vi "Get Subtype Description.vi"(8 "error in (no error)":errorcluster, 11 "Keyboard Action in":refnum<class "Keyboard Action.lvclass">) -> (0 "error out":errorcluster, 2 "Subtype Description":string, 3 "Keyboard Action out":refnum<class "Keyboard Action.lvclass">)   [LabVIEW 2020, in "MacroAssert.lvlib" / "Keyboard Action.lvclass"]
doc: "Gets the subtype description for <B>Step in</B>, which describes what the step's subtype does specifically."
uses:
  Keyboard Action.lvclass
  Keyboard Action.lvclass/Keyboard Action.ctl
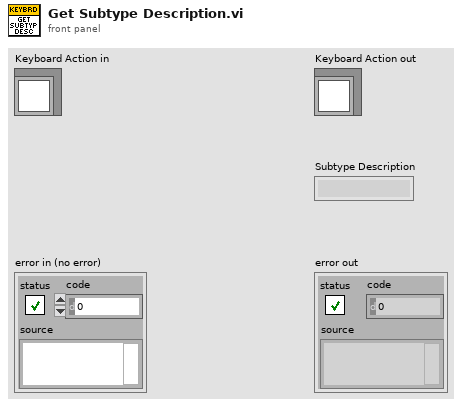
[diagram p1: front panel]
types:
  T1 = typedef "MacroAssert.lvlib/Keyboard Action.lvclass/Keyboard Action Type.ctl" = enum16{"Key Press", "Key Down", "Key Up", "Key Sequence"}
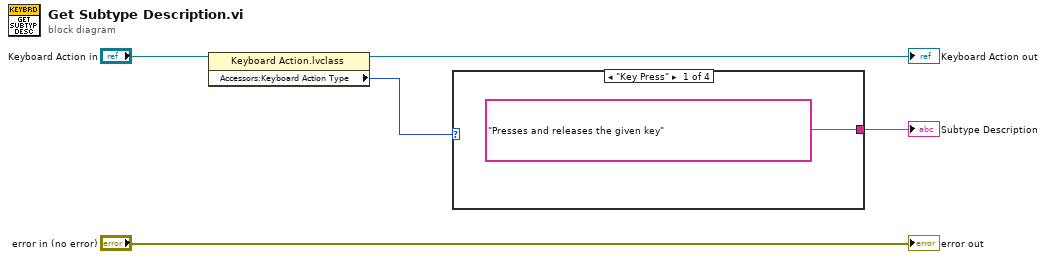
[diagram p0: block diagram]
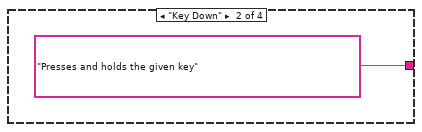
[diagram p2: hidden frame]
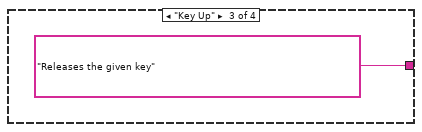
[diagram p3: hidden frame]
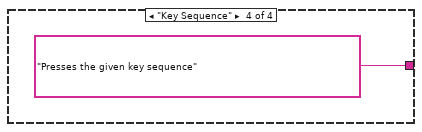
[diagram p4: hidden frame]
diagram:
  n1 = property class="Keyboard Action.lvclass"(reference="Keyboard Action in") -> (reference out=→"Keyboard Action out":refnum<class "Keyboard Action.lvclass">, "Accessors:Keyboard Action Type"=w5:T1)  [unwired: 1 in, 1 out]
  n2 = case shown="\"Key Press\"" w5 {
    tunnel: ["Presses and releases the given key" "Presses and holds the given key" "Releases the given key" "Presses the given key sequence"] -> w1
    frame "Key Press" {
    }
    frame "Key Down" {
    }
    frame "Key Up" {
    }
    frame "Key Sequence" {
    }
  }
  "Subtype Description" <- w1
  "error out" <- "error in (no error)"
